vi "event_global.vi"() -> ()   [LabVIEW 2023]
uses:
  global.vi
panel:
  out "Array 2":bool[](array[boolean])
  in  "operation":enum16{"AND", "OR", "XOR"}(ring)
  out "Boolean 48":bool
  out "Boolean 47":bool
  out "Boolean 46":bool
  out "Boolean 45":bool
  out "Boolean 44":bool
  out "Boolean 43":bool
  out "Boolean 42":bool
  out "Boolean 41":bool
  in  "Boolean 40":bool
  in  "Boolean 39":bool
  in  "Boolean 38":bool
  in  "Boolean 37":bool
  in  "Boolean 36":bool
  in  "Boolean 35":bool
  in  "Boolean 34":bool
  in  "Boolean 33":bool
  in  "Boolean 32":bool
  in  "Boolean 31":bool
  in  "Boolean 30":bool
  in  "Boolean 29":bool
  in  "Boolean 28":bool
  in  "Boolean 27":bool
  in  "Boolean 26":bool
  in  "Boolean 25":bool
  in  "check":bool
  in  "stop":bool
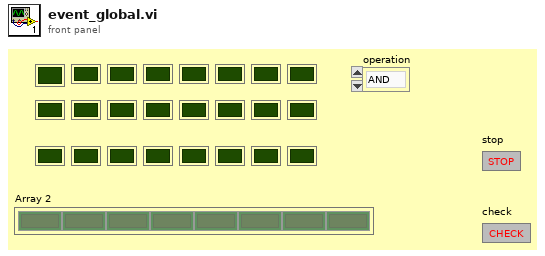
[diagram p1: front panel]
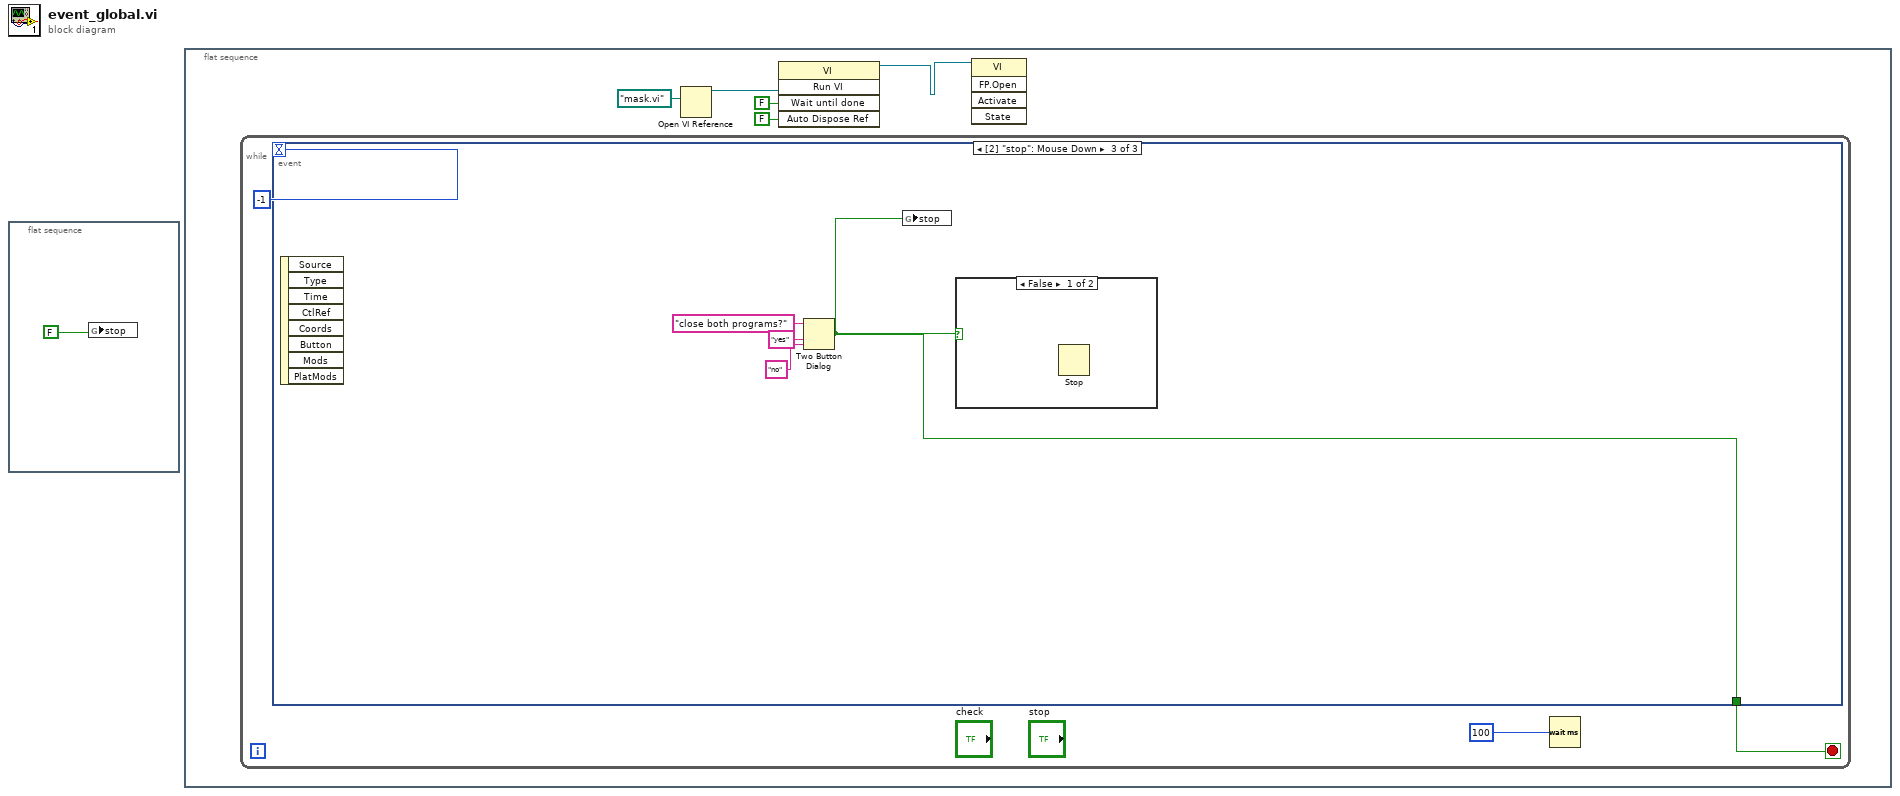
[diagram p0: block diagram]
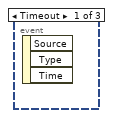
[diagram p2: hidden frame]
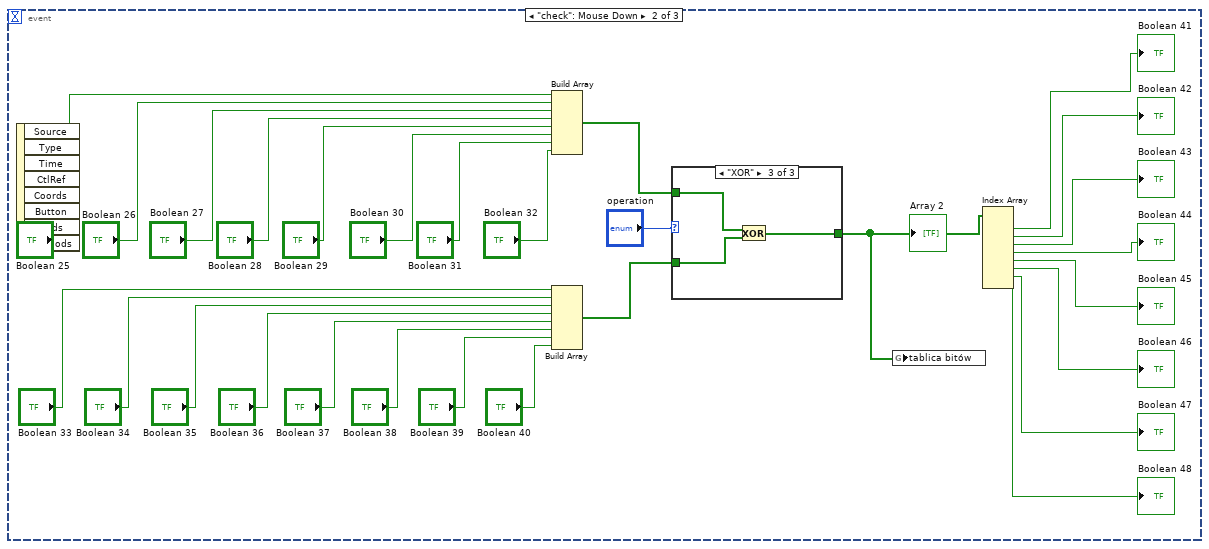
[diagram p3: hidden frame]
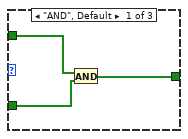
[diagram p4: hidden frame]
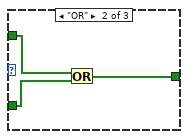
[diagram p5: hidden frame]
diagram:
  n1 = flat-sequence {
    frame #0 {
      n2 = global write "global.vi" "stop"(FALSE) -> ()
    }
  }
  n3 = flat-sequence {
    frame #0 {
      n4 = while {
        stop <- w7 stop-if-true
        n5 = event shown="[2] \"stop\": Mouse Down" {
          selector: _ -> [_ _ _]
          dyn-events: _ -> [_ _ _]
          timeout: -1 -> [_ _ _]
          tunnel: [_ _ w47] -> w7
          event Timeout {
            n6 = event-data() -> ()  [unwired: 1 in, 3 out]
          }
          event "check": Mouse Down {
            n7 = event-data() -> ()  [unwired: 1 in, 8 out]
            n8 = Build Array("Boolean 25", "Boolean 26", "Boolean 27", "Boolean 28", "Boolean 29", "Boolean 30", "Boolean 31", "Boolean 32") -> (w19:bool[])
            n9 = Build Array("Boolean 33", "Boolean 34", "Boolean 35", "Boolean 36", "Boolean 37", "Boolean 38", "Boolean 39", "Boolean 40") -> (w20:bool[])
            n10 = case shown="\"XOR\"" "operation" {
              tunnel: w20 -> [w39 w43 w45]
              tunnel: w19 -> [w40 w42 w46]
              tunnel: [w38 w41 w44] -> w10
              frame "AND", Default {
                n11 = And(x=w40, y=w39) -> (x .and. y?=w38:bool[])
              }
              frame "OR" {
                n12 = Or(x=w42, y=w43) -> (x .or. y?=w41:bool[])
              }
              frame "XOR" {
                n13 = Exclusive Or(1:w45, 2:w46) -> (0:w44:bool[])
              }
            }
            "Array 2" <- w10
            n14 = global write "global.vi" "tablica bitów"(w10) -> ()
            n15 = Index Array(array=w10) -> (element #1=→"Boolean 41":bool, element #2=→"Boolean 42":bool, element #3=→"Boolean 43":bool, element #4=→"Boolean 44":bool, element #5=→"Boolean 45":bool, element #6=→"Boolean 46":bool, element #7=→"Boolean 47":bool, element #8=→"Boolean 48":bool)  [unwired: 8 in]
          }
          event "stop": Mouse Down {
            n16 = event-data() -> ()  [unwired: 1 in, 8 out]
            n17 = Two Button Dialog(message="close both programs?", 1:"no" ("F button name (\"Cancel\")"), 2:"yes" ("T button name (\"OK\")")) -> (T button?=w47:bool)
            n18 = global write "global.vi" "stop"(w47) -> ()
            n19 = case shown="False" w47 {
              frame False {
                n20 = Stop() -> ()  [unwired: 1 in]
              }
              frame True {
              }
            }
          }
        }
        n21 = Wait (ms)(milliseconds to wait=100) -> ()  [unwired: 1 out]
      }
      n22 = Open VI Reference(vi path=path "mask.vi") -> (vi reference=w5:refnum<vi>)  [unwired: 5 in, 1 out]
      n23 = invoke class="VI" method="Run VI"(reference=w5, "Wait until done"=FALSE ("Wait Until Done"), "Auto Dispose Ref"=FALSE ("Auto Dispose Reference")) -> (reference out=w2:refnum<vi>)  [unwired: 2 in, 4 out]
      n24 = invoke class="VI" method="FP.Open"(reference=w2) -> ()  [unwired: 4 in, 5 out]
    }
  }
